vi "Subvi_converter_Craig_to_Jonas.vi"(1 "array":dbl[](array[numeric])) -> (0 "appended array":dbl[](array[numeric]))   [LabVIEW 2017]
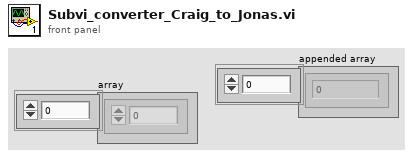
[diagram p1: front panel]
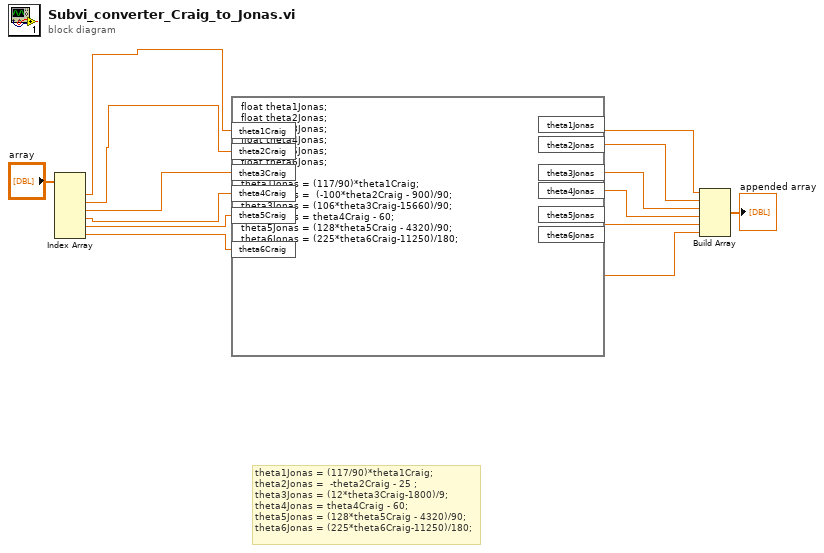
[diagram p0: block diagram]
diagram:
  # "theta1Jonas = (117/90)*theta1Craig;\ntheta2Jonas =  -theta2Craig - 25 ;\ntheta3Jonas = (12*theta3Craig-1800)/9;\ntheta4Jonas = theta4Craig - 60;\ntheta5Jonas = (128*theta5Craig - 4320)/90;\ntheta6Jonas = (225*theta6Craig-11250)/180;"
  n1 = Index Array(array="array") -> (element #1=w13:dbl, element #2=w12:dbl, element #3=w11:dbl, element #4=w10:dbl, element #5=w9:dbl, element #6=w8:dbl)  [unwired: 6 in]
  n2 = formula code="float theta1Jonas;\nfloat theta2Jonas;\nfloat theta3Jonas;\nfloat theta4Jonas;\nfloat theta5Jonas;\nfloat theta6Jonas;\n\ntheta1Jonas = (117/90)*theta1Craig;\ntheta2Jonas =  (-100*theta2Craig - 900)/90;\ntheta3Jonas = (106*theta3Craig-15660)/90;\ntheta4Jonas = theta4Craig - 60;\ntheta5Jonas = (128*theta5Craig - 4320)/90;\ntheta6Jonas = (225*theta6Craig-11250)/180;"("theta1Craig"=w13, "theta3Craig"=w11, "theta4Craig"=w10, "theta5Craig"=w9, "theta6Craig"=w8, "theta2Craig"=w12) -> ("theta1Jonas"=w7:dbl, "theta2Jonas"=w6:dbl, "theta3Jonas"=w5:dbl, "theta4Jonas"=w4:dbl, "theta5Jonas"=w3:dbl, "theta6Jonas"=w2:dbl)
  n3 = Build Array(w7, w6, w5, w4, w3, w2) -> (→"appended array":dbl[])
